vi "Write RT FIFO.vi"(6 "overwrite on timeout (T)":bool, 7 "fifo options":T1, 8 "error in (no error)":errorcluster, 9 "timeout in ms (0)":i32, 10 "element":u8[](array[numeric]), 11 "rt fifo in":refnum<k33>) -> (0 "error out":errorcluster, 1 "timed out?":bool, 3 "rt fifo out":refnum<k33>, 4 "# elements":u32)   [LabVIEW 2021, in "DSF Core.lvlib" / "Interface.lvclass"]
uses:
  Interface.lvclass
  Typedefs/DSF FIFO Options.ctl
  Framework/Framework.lvclass
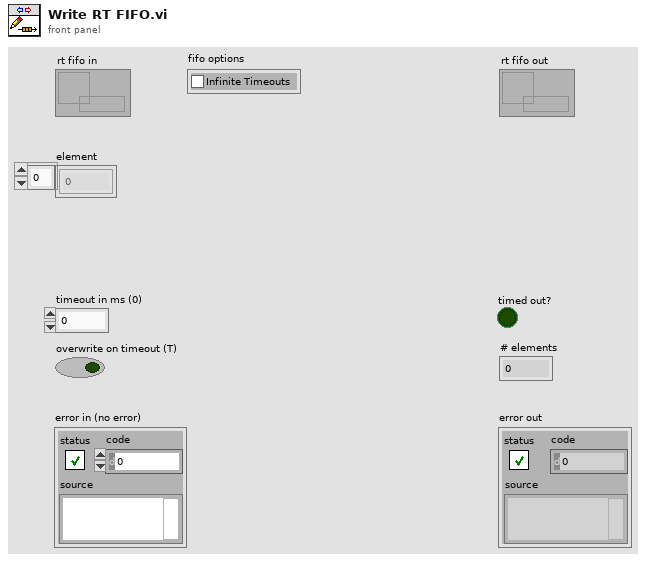
[diagram p1: front panel]
types:
  T1 = typedef "DSF Core.lvlib/Framework.lvclass/DSF FIFO Options.ctl" = cluster{"Infinite Timeouts":bool}
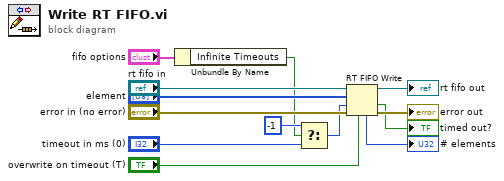
[diagram p0: block diagram]
diagram:
  n1 = Unbundle By Name("fifo options") -> ("Infinite Timeouts"=w1:bool)
  n2 = Select(t=-1, s=w1, f="timeout in ms (0)") -> (s? t:f=w7:i32)
  n3 = RT FIFO Write(0:"rt fifo in", 1:"element", 2:w7, 3:"error in (no error)", 5:"overwrite on timeout (T)") -> (7:→"# elements":u32, 8:→"rt fifo out":refnum<k33>, 10:→"timed out?":bool, 11:→"error out":errorcluster)
